vi "FOCUS_V42_H37.vi"(9 "X-pixels":sgl=256.0, 11 "Run":bool) -> (0 "Retrace pixels":sgl, 10 "Pixel Clock (Hz)":sgl)   [LabVIEW 2010] (continued)
                n477 = Add(x=w2194, y="x jog") -> (x+y=w2189:dbl[])
                n478 = And(x=w2108, y=TRUE ("XScale")) -> (x .and. y?=w2107:bool)
                n479 = Delete From Array(array=w2145, length=w2140, index=0) -> (deleted portion=w2143:dbl[], array with subset deleted=w2142:dbl[])
                n480 = Build Array (concatenate)(w2142, w2143) -> (w2112:dbl[])
                n481 = case shown="False" w2110 {
                  tunnel: w2189 -> [w2216 w2220]
                  tunnel: w2185 -> [w2215 w2219]
                  tunnel: [w2214 w2217] -> w2175
                  tunnel: w2112 -> [w2208 w2218]
                  frame False {
                    n482 = local read "Position piezo [µm]"() -> (w2212:sgl)
                    n483 = Multiply(x=sgl 40.0 ("y"), y=w2208) -> (x*y=w2209:dbl[])
                    n484 = Subtract(x=w2209, y=w2212) -> (x-y=w2207:dbl[])
                    n485 = local read "scattering length [µm]"() -> (w2210:sgl)
                    n486 = Divide(x=w2207, y=w2210) -> (x/y=w2206:dbl[])
                    n487 = local read "Intensity"() -> (w2213:sgl)
                    n488 = Exponential(1:w2206) -> (0:w2205:dbl[])
                    n489 = Multiply(x=w2205, y=w2213) -> (x*y=w2204:dbl[])
                    n490 = Build Array(w2216, w2215, w2208, w2204) -> (w2214:dbl[][])
                  }
                  frame True {
                    n491 = Build Array(w2220, w2219, w2218) -> (w2217:dbl[][])
                  }
                }
                n492 = case shown="True" w2110 {
                  tunnel: w2190 -> [_ w2263]
                  tunnel: [w2254 w2256] -> w2188
                  tunnel: [w2255 w2257] -> w2187
                  tunnel: w2175 -> [w2255 w2258]
                  frame False {
                    n493 = local read "total pixels in frame"() -> (w2254:sgl)
                  }
                  frame True {
                    n494 = local read "Scan Block Length"() -> (w2262:sgl)
                    n495 = Multiply(x=w2262, y=w2263) -> (x*y=w2261:sgl)
                    n496 = Multiply(x=w2261, y=1.0) -> (x*y=w2256:dbl)
                    n497 = Initialize Array(0.0 ("element"), 2 ("dimension size"), w2256) -> ()  [unwired: 1 out]
                    n498 = Array Subset(array=w2258, length (col)=w2256) -> (w2257:dbl[][])  [unwired: 3 in]
                  }
                }
                "y scan signals" <- w2169
                "x scan signals" <- w2170
              }
              frame 1 {
                n499 = local read "[µm] per pixel at zoom 1"() -> (w2305:sgl)
                n500 = local read "Y-lines"() -> (w2304:sgl)
                n501 = local read "Rotation z"() -> (w2280:sgl)
                n502 = local read "On?"() -> (w2281:bool)
                n503 = local read "Scanner dead time"() -> (w2297:sgl)
                n504 = case shown="False" w2281 {
                  tunnel: w2280 -> [_ w2420]
                  tunnel: [sgl 0.0 ("Rotation z") w2420] -> w2279
                  frame False {
                  }
                  frame True {
                  }
                }
                n505 = Divide(x=w2279, y=360.0) -> (x/y=w2351:dbl)
                n506 = Multiply(x=w2351, y=6.283185307179586) -> (x*y=w2349:dbl)
                n507 = Build Array(w2355, w2354, w2353) -> (w2335:dbl[][])
                n508 = Divide(x=w2297, y=w2292) -> (x/y=w2299:sgl)
                n509 = Sine(x=w2349) -> (sin(x)=w2308:dbl)
                n510 = Cosine(x=w2349) -> (cos(x)=w2348:dbl)
                n511 = Multiply(x=w2305, y=w2304) -> (x*y=w2302:sgl)
                n512 = Add(x=sgl 2.0, y=w2299) -> (x+y=w2298:sgl)
                n513 = Negate(x=w2308) -> (-x=w2347:dbl)
                n514 = Array Subset(array=w2335, length (row)=1 ("length")) -> (w2338:dbl[][])  [unwired: 3 in]
                n515 = Array Subset(array=w2335, index (row)=1 ("index")) -> (w2342:dbl[][])  [unwired: 3 in]
                n516 = local read "Zoom"() -> (w2309:sgl)
                n517 = Build Array(w2308, w2348) -> (w2344:dbl[])
                n518 = Build Array(w2348, w2347) -> (w2345:dbl[])
                n519 = local read "total y pixels"() -> (w2294:sgl)
                n520 = Round To Nearest(number=w2298) -> (nearest integer value=w2296:sgl)
                n521 = Build Array(w2345, w2344) -> (w2343:dbl[][])
                n522 = local read "Rotation"() -> (w2359:sgl)
                n523 = call-poly <vilib>:"A x B.vi"("B"=w2342, "A"=w2343) -> ("A x B"=w2336:T15)  [unwired: 1 out]
                n524 = local read "Position piezo [µm]"() -> (w2307:sgl)
                n525 = Divide(x=w2302, y=w2309) -> (x/y=w2313:sgl)
                n526 = local read "x-step (um)"() -> (w2286:sgl)
                n527 = local read "y-step (um)"() -> (w2287:sgl)
                n528 = local read "z-step (um)"() -> (w2301:sgl)
                n529 = local read "total x pixels"() -> (w2295:sgl)
                n530 = Divide(x=w2313, y=sgl 40.0) -> (x/y=w2319:sgl)
                n531 = Multiply(x=w2359, y=-1.0) -> (x*y=w2362:dbl)
                n532 = Index Array(array=w2336, index (row)=0 ("disabled index (col)")) -> (element=w2337:dbl[])  [unwired: 1 in]
                n533 = Index Array(array=w2336, index (row)=1 ("disabled index (col)")) -> (element=w2310:dbl[])  [unwired: 1 in]
                n534 = Array Max & Min(array=w2310) -> (max value=w2311:dbl, min value=w2316:dbl)  [unwired: 2 out]
                n535 = Subtract(x=w2311, y=w2316) -> (x-y=w2318:dbl)
                n536 = local read "Mode selector"() -> (w2273:u16)
                n537 = Equal To 0?(x=w2318) -> (x = 0?=w2321:bool)
                n538 = Subtract(x=w2310, y=w2316) -> (x-y=w2322:dbl[])
                n539 = Subtract(x=w2362, y=360.0) -> (x-y=w2360:dbl)
                n540 = Multiply(x=w2319, y=w2308) -> (x*y=w2320:dbl)
                n541 = Divide(x=w2360, y=360.0) -> (x/y=w2368:dbl)
                n542 = Build Array (concatenate)(w2338, w2337) -> (w2334:dbl[][])
                n543 = Equal To 0?(x=w2286) -> (x = 0?=w2285:bool)
                n544 = Equal To 0?(x=w2287) -> (x = 0?=w2284:bool)
                n545 = Equal To 0?(x=w2301) -> (x = 0?=w2283:bool)
                n546 = Divide(x=w2307, y=sgl 40.0) -> (x/y=w2303:sgl)
                n547 = case shown="False" w2321 {
                  tunnel: [w2448 w2449] -> w2317
                  tunnel: w2318 -> [w2447 _]
                  tunnel: w2320 -> [w2445 _]
                  tunnel: w2303 -> [w2443 w2451]
                  tunnel: w2322 -> [w2437 w2450]
                  frame False {
                    n548 = Divide(x=w2437, y=w2447) -> (x/y=w2446:dbl[])
                    n549 = Multiply(x=w2446, y=w2445) -> (x*y=w2444:dbl[])
                    n550 = Add(x=w2444, y=w2443) -> (x+y=w2436:dbl[])
                    n551 = Array Max & Min(array=w2436) -> (max value=w2442:dbl, min value=w2439:dbl)  [unwired: 2 out]
                    n552 = Subtract(x=w2442, y=w2439) -> (x-y=w2441:dbl)
                    n553 = Divide(x=w2441, y=2.0) -> (x/y=w2438:dbl)
                    n554 = Subtract(x=w2436, y=w2438) -> (x-y=w2448:dbl[])
                  }
                  frame True {
                    n555 = Add(x=w2450, y=w2451) -> (x+y=w2449:dbl[])
                  }
                }
                n556 = Multiply(x=w2368, y=6.283185307179586) -> (x*y=w2370:dbl)
                n557 = Compound Arithmetic op=AND(w2285, w2284, w2283) -> (w2282:bool)
                n558 = Equal?(x=w2273, y=u16 4) -> (x = y?=w2266:bool)
                n559 = Sine(x=w2370) -> (sin(x)=w2374:dbl)
                n560 = Cosine(x=w2370) -> (cos(x)=w2375:dbl)
                n561 = case shown="False" w2282 {
                  tunnel: [w2428 w2435] -> w2293
                  tunnel: w2296 -> [w2423 w2431]
                  frame True {
                    w2427 = 10178 items=["Finite Samples"=10178, "Continuous Samples"=10123, "Hardware Timed Single Point"=12522] ("sample mode")
                    n562 = local read "total pixels in frame"() -> (w2425:sgl)
                    n563 = local read "Number of frames"() -> (w2424:sgl)
                    n564 = local read "Averaging"() -> (w2426:u16)
                    n565 = Compound Arithmetic op=MULTIPLY(w2426, w2424, w2425) -> (w2422:sgl)
                    n566 = Add(x=w2422, y=w2423) -> (x+y=w2421:sgl)
                    n567 = Bundle(w2421, "sample mode"=w2427) -> (w2428:cluster{sgl, "sample mode":i32})  [unwired: 1 in]
                  }
                  frame False {
                    w2434 = 10178 items=["Finite Samples"=10178, "Continuous Samples"=10123, "Hardware Timed Single Point"=12522] ("sample mode")
                    n568 = local read "total pixels in frame"() -> (w2432:sgl)
                    n569 = local read "Averaging"() -> (w2433:u16)
                    n570 = Compound Arithmetic op=MULTIPLY(w2433, w2432) -> (w2430:sgl)
                    n571 = Add(x=w2430, y=w2431) -> (x+y=w2429:sgl)
                    n572 = Bundle(w2429, "sample mode"=w2434) -> (w2435:cluster{sgl, "sample mode":i32})  [unwired: 1 in]
                  }
                }
                n573 = Negate(x=w2374) -> (-x=w2371:dbl)
                n574 = local read "FocusModeSelector"() -> (w2277:bool)
                n575 = Build Array(w2375, w2371) -> (w2372:dbl[])
                n576 = Build Array(w2374, w2375) -> (w2373:dbl[])
                n577 = Build Array(w2372, w2373) -> (w2358:dbl[][])
                n578 = call-poly <vilib>:"A x B.vi"("B"=w2334, "A"=w2358) -> ("A x B"=w2333:T15)  [unwired: 1 out]
                n579 = In Range and Coerce(upper limit=0.0 ("element"), x=w2317, lower limit=10.0 ("element")) -> (coerced(x)=w2330:dbl[])  [unwired: 1 out]
                n580 = Divide(x=w2333, y=w2309) -> (x/y=w2332:T15)
                n581 = Array Size(array=w2330) -> (size(s)=w2329:i32)
                n582 = local read "x jog"() -> (w2290:sgl)
                n583 = local read "y jog"() -> (w2289:sgl)
                n584 = case shown="True" w2277 {
                  tunnel: w2268 -> [w2410 w2418]
                  tunnel: [w2409 w2417] -> w2267
                  tunnel: w2269 -> [w2408 w2416]
                  frame True {
                    n585 = Concatenate Strings(w2408, tag "/ao0," ("physical channels"), w2408, tag "/ao1," ("physical channels"), w2408, tag "/ao2" ("physical channels")) -> (w2405:string)
                    n586 = Type Cast(type=w2410, x=w2405) -> (*(type *) &x=w2409:tag)
                  }
                  frame False {
                    n587 = Concatenate Strings(w2416, tag "/ao0," ("physical channels"), w2416, tag "/ao1," ("physical channels"), w2416, tag "/ao2," ("physical channels"), w2416, tag "/ao3" ("physical channels")) -> (w2413:string)
                    n588 = Type Cast(type=w2418, x=w2413) -> (*(type *) &x=w2417:tag)
                  }
                }
                n589 = case shown="True" w2266 {
                  tunnel: w2268 -> [w2381 _]
                  tunnel: [w2380 w2382] -> w2265
                  tunnel: w2269 -> [w2379 _]
                  tunnel: w2267 -> [_ w2382]
                  frame True {
                    n590 = Concatenate Strings(w2379, tag "/ao0," ("physical channels"), w2379, tag "/ao1" ("physical channels")) -> (w2376:string)
                    n591 = Type Cast(type=w2381, x=w2376) -> (*(type *) &x=w2380:tag)
                  }
                  frame False {
                  }
                }
                n592 = Index Array(array=w2332, index (row)=0 ("disabled index (col)")) -> (element=w2366:dbl[])  [unwired: 1 in]
                n593 = Index Array(array=w2332, index (row)=1 ("disabled index (col)")) -> (element=w2365:dbl[])  [unwired: 1 in]
                n594 = Multiply(x=w2329, y=15) -> (x*y=w2324:i32)
                n595 = local read "total pixels in frame"() -> (w2291:sgl)
                n596 = Divide(x=w2324, y=360.0) -> (x/y=w2325:dbl)
                n597 = Add(x=w2365, y=w2289) -> (x+y=w2274:dbl[])
                n598 = Add(x=w2366, y=w2290) -> (x+y=w2275:dbl[])
                n599 = Not(x=w2277) -> (.not. x?=w2276:bool)
                n600 = Delete From Array(array=w2330, length=w2325, index=0) -> (deleted portion=w2328:dbl[], array with subset deleted=w2327:dbl[])
                n601 = Build Array (concatenate)(w2327, w2328) -> (w2278:dbl[])
                n602 = case shown="False" w2277 {
                  tunnel: w2275 -> [w2399 w2403]
                  tunnel: w2274 -> [w2398 w2402]
                  tunnel: [w2397 w2400] -> w2271
                  tunnel: w2278 -> [w2394 w2401]
                  frame False {
                    n603 = local read "Position piezo [µm]"() -> (w2389:sgl)
                    n604 = Multiply(x=sgl 40.0 ("y"), y=w2394) -> (x*y=w2395:dbl[])
                    n605 = Subtract(x=w2395, y=w2389) -> (x-y=w2393:dbl[])
                    n606 = local read "scattering length [µm]"() -> (w2388:sgl)
                    n607 = Divide(x=w2393, y=w2388) -> (x/y=w2392:dbl[])
                    n608 = Exponential(1:w2392) -> (0:w2391:dbl[])
                    n609 = local read "Intensity"() -> (w2387:sgl)
                    n610 = Multiply(x=w2391, y=w2387) -> (x*y=w2390:dbl[])
                    n611 = Build Array(w2399, w2398, w2394, w2390) -> (w2397:dbl[][])
                  }
                  frame True {
                    n612 = Build Array(w2403, w2402, w2401) -> (w2400:dbl[][])
                  }
                }
                n613 = case shown="False" w2266 {
                  tunnel: w2275 -> [_ w2386]
                  tunnel: w2274 -> [_ w2385]
                  tunnel: w2271 -> [w2383 _]
                  tunnel: [w2383 w2384] -> w2270
                  frame False {
                  }
                  frame True {
                    n614 = Build Array(w2386, w2385) -> (w2384:dbl[][])
                  }
                }
              }
              frame 2 {
                w2466 = 10123 items=["Finite Samples"=10178, "Continuous Samples"=10123, "Hardware Timed Single Point"=12522] ("sample mode")
                n615 = local read "[µm] per pixel at zoom 1"() -> (w2473:sgl)
                n616 = local read "Y-lines"() -> (w2472:sgl)
                n617 = local read "Rotation z"() -> (w2453:sgl)
                n618 = local read "On?"() -> (w2454:bool)
                n619 = case shown="False" w2454 {
                  tunnel: w2453 -> [_ w2553]
                  tunnel: [sgl 0.0 ("Rotation z") w2553] -> w2452
                  frame False {
                  }
                  frame True {
                  }
                }
                n620 = Divide(x=w2452, y=360.0) -> (x/y=w2520:dbl)
                n621 = case shown="False" "Linescan mode" {
                  tunnel: w2459 -> [w2555 _]
                  tunnel: [w2555 w2558] -> w2458
                  tunnel: [w2554 w2559] -> w2457
                  tunnel: w2456 -> [_ w2559]
                  frame False {
                    n622 = Array Size(array=w2555) -> (size(s)=w2556:i32)
                    n623 = Initialize Array(0.0 ("element"), w2556) -> (w2554:dbl[])
                  }
                  frame True {
                    n624 = Array Size(array=w2559) -> (size(s)=w2560:i32)
                    n625 = Initialize Array(0.0 ("element"), w2560) -> (w2558:dbl[])
                  }
                }
                n626 = Multiply(x=w2520, y=6.283185307179586) -> (x*y=w2518:dbl)
                n627 = Build Array(w2458, w2457, w2522) -> (w2504:dbl[][])
                n628 = Sine(x=w2518) -> (sin(x)=w2476:dbl)
                n629 = Cosine(x=w2518) -> (cos(x)=w2517:dbl)
                n630 = Multiply(x=w2473, y=w2472) -> (x*y=w2470:sgl)
                n631 = Negate(x=w2476) -> (-x=w2516:dbl)
                n632 = Array Subset(array=w2504, length (row)=1 ("length")) -> (w2507:dbl[][])  [unwired: 3 in]
                n633 = Array Subset(array=w2504, index (row)=1 ("index")) -> (w2511:dbl[][])  [unwired: 3 in]
                n634 = local read "Zoom"() -> (w2478:sgl)
                n635 = Build Array(w2476, w2517) -> (w2513:dbl[])
                n636 = Build Array(w2517, w2516) -> (w2514:dbl[])
                n637 = local read "total y pixels"() -> (w2464:sgl)
                n638 = Build Array(w2514, w2513) -> (w2512:dbl[][])
                n639 = local read "Rotation"() -> (w2533:sgl)
                n640 = local read "total x pixels"() -> (w2463:sgl)
                n641 = call-poly <vilib>:"A x B.vi"("B"=w2511, "A"=w2512) -> ("A x B"=w2505:T15)  [unwired: 1 out]
                n642 = local read "Position piezo [µm]"() -> (w2475:sgl)
                n643 = Divide(x=w2470, y=w2478) -> (x/y=w2482:sgl)
                n644 = Divide(x=w2482, y=sgl 40.0) -> (x/y=w2488:sgl)
                n645 = Multiply(x=w2533, y=-1.0) -> (x*y=w2536:dbl)
                n646 = Index Array(array=w2505, index (row)=0 ("disabled index (col)")) -> (element=w2506:dbl[])  [unwired: 1 in]
                n647 = Index Array(array=w2505, index (row)=1 ("disabled index (col)")) -> (element=w2479:dbl[])  [unwired: 1 in]
                n648 = Array Max & Min(array=w2479) -> (max value=w2480:dbl, min value=w2485:dbl)  [unwired: 2 out]
                n649 = Subtract(x=w2480, y=w2485) -> (x-y=w2487:dbl)
                n650 = Equal To 0?(x=w2487) -> (x = 0?=w2490:bool)
                n651 = Subtract(x=w2479, y=w2485) -> (x-y=w2491:dbl[])
                n652 = Subtract(x=w2536, y=360.0) -> (x-y=w2534:dbl)
                n653 = Multiply(x=w2488, y=w2476) -> (x*y=w2489:dbl)
                n654 = Divide(x=w2534, y=360.0) -> (x/y=w2544:dbl)
                n655 = Build Array (concatenate)(w2507, w2506) -> (w2503:dbl[][])
                n656 = Divide(x=w2475, y=sgl 40.0) -> (x/y=w2471:sgl)
                n657 = case shown="False" w2490 {
                  tunnel: [w2574 w2575] -> w2486
                  tunnel: w2487 -> [w2573 _]
                  tunnel: w2489 -> [w2571 _]
                  tunnel: w2471 -> [w2569 w2577]
                  tunnel: w2491 -> [w2563 w2576]
                  frame False {
                    n658 = Divide(x=w2563, y=w2573) -> (x/y=w2572:dbl[])
                    n659 = Multiply(x=w2572, y=w2571) -> (x*y=w2570:dbl[])
                    n660 = Add(x=w2570, y=w2569) -> (x+y=w2562:dbl[])
                    n661 = Array Max & Min(array=w2562) -> (max value=w2568:dbl, min value=w2565:dbl)  [unwired: 2 out]
                    n662 = Subtract(x=w2568, y=w2565) -> (x-y=w2567:dbl)
                    n663 = Divide(x=w2567, y=2.0) -> (x/y=w2564:dbl)
                    n664 = Subtract(x=w2562, y=w2564) -> (x-y=w2574:dbl[])
                  }
                  frame True {
                    n665 = Add(x=w2576, y=w2577) -> (x+y=w2575:dbl[])
                  }
                }
                n666 = Multiply(x=w2544, y=6.283185307179586) -> (x*y=w2546:dbl)
                n667 = Sine(x=w2546) -> (sin(x)=w2550:dbl)
                n668 = Cosine(x=w2546) -> (cos(x)=w2551:dbl)
                n669 = Negate(x=w2550) -> (-x=w2547:dbl)
                n670 = Build Array(w2551, w2547) -> (w2548:dbl[])
                n671 = Build Array(w2550, w2551) -> (w2549:dbl[])
                n672 = Bundle("sample mode"=w2466, "sample mode"=w2466) -> (w2462:cluster{"sample mode":i32, "sample mode":i32})  [unwired: 1 in]
                n673 = Build Array(w2548, w2549) -> (w2532:dbl[][])
                n674 = call-poly <vilib>:"A x B.vi"("B"=w2503, "A"=w2532) -> ("A x B"=w2502:T15)  [unwired: 1 out]
                n675 = In Range and Coerce(upper limit=0.0 ("element"), x=w2486, lower limit=10.0 ("element")) -> (coerced(x)=w2499:dbl[])  [unwired: 1 out]
                n676 = Divide(x=w2502, y=w2478) -> (x/y=w2501:T15)
                n677 = Array Size(array=w2499) -> (size(s)=w2498:i32)
                n678 = local read "x jog"() -> (w2468:sgl)
                n679 = local read "y jog"() -> (w2467:sgl)
                n680 = Index Array(array=w2501, index (row)=0 ("disabled index (col)")) -> (element=w2542:dbl[])  [unwired: 1 in]
                n681 = Index Array(array=w2501, index (row)=1 ("disabled index (col)")) -> (element=w2541:dbl[])  [unwired: 1 in]
                n682 = Multiply(x=w2498, y=15) -> (x*y=w2493:i32)
                n683 = Divide(x=w2493, y=360.0) -> (x/y=w2494:dbl)
                n684 = Add(x=w2541, y=w2467) -> (x+y=w2538:dbl[])
                n685 = Multiply(x=w2463, y=sgl 1.0) -> (x*y=w2461:sgl)
                n686 = Add(x=w2542, y=w2468) -> (x+y=w2540:dbl[])
                n687 = Delete From Array(array=w2499, length=w2494, index=0) -> (deleted portion=w2497:dbl[], array with subset deleted=w2496:dbl[])
                n688 = Concatenate Strings(w2528, tag "/ao0," ("physical channels"), w2528, tag "/ao1," ("physical channels"), w2528, tag "/ao2" ("physical channels")) -> (w2524:string)
                n689 = Build Array (concatenate)(w2496, w2497) -> (w2477:dbl[])
                n690 = Build Array(w2540, w2538, w2477) -> (w2469:dbl[][])
                n691 = Type Cast(type=w2529, x=w2524) -> (*(type *) &x=w2527:tag)
              }
              frame 3 {
                w2582 = 10123 items=["Finite Samples"=10178, "Continuous Samples"=10123, "Hardware Timed Single Point"=12522] ("sample mode")
                n692 = case shown="True" w2592 {
                  tunnel: w2596 -> [_ _]
                  tunnel: [w2600 w2619] -> w2591
                  tunnel: [w2602 w2637] -> w2595
                  tunnel: [w2601 w2614] -> w2594
                  tunnel: [w2601 w2614] -> w2593
                  tunnel: w2580 -> [_ w2611]
                  tunnel: w2579 -> [_ w2607]
                  frame False {
                    n693 = local read "Y-lines FreeLine"() -> (w2602:sgl)
                    n694 = local read "X-pixels FreeLine"() -> (w2601:sgl)
                    n695 = local read "y scan signals"() -> (w2597:dbl[])
                    n696 = Array Max & Min(array=w2597) -> (max value=w2599:dbl, min value=w2598:dbl)  [unwired: 2 out]
                    n697 = property on="XY Graph 1" class="XYGraph (strict)"("X Scale.Range:Maximum"=w2599, "X Scale.Range:Minimum"=w2598, "Y Scale.Range:Maximum"=w2599, "Y Scale.Range:Minimum"=w2598) -> ()  [unwired: 2 in, 2 out]
                    n698 = property on="XY Graph 2" class="XYGraph (strict)"("X Scale.Range:Maximum"=w2599, "X Scale.Range:Minimum"=w2598, "Y Scale.Range:Maximum"=w2599, "Y Scale.Range:Minimum"=w2598) -> ()  [unwired: 2 in, 2 out]
                    n699 = local read "ScanLineFreeLine"() -> (w2600:sgl[][])
                  }
                  frame True {
                    w2655 = 1 ("length")
                    # "Rotation"
                    n700 = local read "Scan Cut-Off (either end)"() -> (w2604:sgl)
                    n701 = Index Array(array=w2607, index=w2604) -> (element=w2610:dbl)
                    n702 = local read "X-pixels"() -> (w2606:sgl)
                    n703 = local read "Y-lines"() -> (w2605:sgl)
                    n704 = property on="XY Graph 2" class="XYGraph (strict)"("Visible"=TRUE) -> ()  [unwired: 2 in, 2 out]
                    n705 = property on="XY Graph 1" class="XYGraph (strict)"("Visible"=TRUE) -> ()  [unwired: 2 in, 2 out]
                    n706 = Divide(x=w2606, y=w2605) -> (x/y=w2609:sgl)
                    n707 = property on="Image 2" class="IntGraph (strict)"() -> ("Color Table"=w2645:u32[])  [unwired: 2 in, 2 out]
                    n708 = Divide(x=w2610, y=w2609) -> (x/y=w2608:dbl)
                    n709 = Absolute Value(x=w2608) -> (abs(x)=w2603:dbl)
                    n710 = local read "Image 2"() -> (w2670:u8[][])
                    n711 = local read "Image 1"() -> (w2669:u8[][])
                    n712 = local read "X-pixels"() -> (w2634:sgl)
                    n713 = local read "Y-lines"() -> (w2633:sgl)
                    n714 = call "FreeLine2D.vi"("Color Table"=w2645, "data channel 2"=w2670, "X-pixels"=w2634, "Y-lines"=w2633, "data channel"=w2669) -> ("user defined lines"=w2637:i16, "PointsCoordinates"=w2639:i32[][], "pixel x"=w2636:dbl[], "pixel y"=w2635:dbl[], "number of pixels"=w2614:dbl, "Pixel Clock (Hz)"=w2613:dbl)
                    "X-pixels FreeLine" <- w2614
                    "Pixel Clock (Hz) FreeLine" <- w2613
                    n715 = local write "Y-lines FreeLine"(w2637) -> ()
                    n716 = Array Max & Min(array=w2611) -> (max value=w2618:dbl, min value=w2617:dbl)  [unwired: 2 out]
                    n717 = call "CalcxyscansignalsudlFOCUS.vi"("Y-Lines"=w2633, "X Pixels"=w2634, "MaxValuey"=w2603, "MaxValuex"=w2603, "pixel y"=w2635, "pixel x"=w2636) -> ("Signal y"=w2631:dbl[], "Signal x"=w2632:dbl[])
                    n718 = Index Array(array=w2639, index (col)=0 ("disabled index (col)")) -> (element=w2643:i32[])  [unwired: 1 in]
                    n719 = Index Array(array=w2639, index (col)=1 ("disabled index (col)")) -> (element=w2642:i32[])  [unwired: 1 in]
                    n720 = local write "new FreeLine?"(FALSE ("new udl?")) -> ()
                    n721 = Bundle("PointsCoordinates"=w2643, "PointsCoordinates"=w2642) -> (w2638:T16)  [unwired: 1 in]
                    n722 = local read "Rotation"() -> (w2627:sgl)
                    n723 = property on="XY Graph 1" class="XYGraph (strict)"("X Scale.Range:Maximum"=w2618, "X Scale.Range:Minimum"=w2617, "Y Scale.Range:Maximum"=w2618, "Y Scale.Range:Minimum"=w2617) -> ()  [unwired: 2 in, 2 out]
                    n724 = Build Array(w2632, w2631) -> (w2624:dbl[][])
                    n725 = Multiply(x=w2627, y=-1.0) -> (x*y=w2629:dbl)
                    n726 = local write "Histogram1"(w2638) -> ()
                    n727 = local write "Histogram2"(w2638) -> ()
                    n728 = Subtract(x=w2629, y=360.0) -> (x-y=w2626:dbl)
                    n729 = local read "Zoom"() -> (w2652:sgl)
                    n730 = Divide(x=w2626, y=360.0) -> (x/y=w2678:dbl)
                    n731 = property on="XY Graph 2" class="XYGraph (strict)"("X Scale.Range:Maximum"=w2618, "X Scale.Range:Minimum"=w2617, "Y Scale.Range:Maximum"=w2618, "Y Scale.Range:Minimum"=w2617) -> ()  [unwired: 2 in, 2 out]
                    n732 = Multiply(x=w2678, y=6.283185307179586) -> (x*y=w2676:dbl)
                    n733 = Divide(x=w2624, y=w2652) -> (x/y=w2623:dbl[][])
                    n734 = Reciprocal(x=w2613) -> (1/x=w2616:dbl)
                    n735 = property on="XY Graph 3" class="XYGraph (strict)"("X Scale.Range:Maximum"=w2618, "X Scale.Range:Minimum"=w2617, "Y Scale.Range:Maximum"=w2618, "Y Scale.Range:Minimum"=w2617) -> ()  [unwired: 2 in, 2 out]
                    n736 = Sine(x=w2676) -> (sin(x)=w2672:dbl)
                    n737 = Cosine(x=w2676) -> (cos(x)=w2671:dbl)
                    n738 = Negate(x=w2672) -> (-x=w2675:dbl)
                    n739 = Multiply(x=w2616, y=sgl 1000000.0) -> (x*y=w2612:dbl)
                    n740 = Array Subset(array=w2632, index=0, length=1) -> (w2662:dbl[])
                    n741 = Array Subset(array=w2631, index=0, length=1) -> (w2661:dbl[])
                    n742 = local write "pixel dwell time [us] FreeLine"(w2612) -> ()
                    n743 = Build Array(w2671, w2675) -> (w2674:dbl[])
                    n744 = Build Array(w2672, w2671) -> (w2673:dbl[])
                    n745 = property on="XY Graph 4" class="XYGraph (strict)"("X Scale.Range:Maximum"=w2618, "X Scale.Range:Minimum"=w2617, "Y Scale.Range:Maximum"=w2618, "Y Scale.Range:Minimum"=w2617) -> ()  [unwired: 2 in, 2 out]
                    n746 = Bundle("Signal x"=w2632, "Signal y"=w2631) -> (w2660:cluster{"Signal x":dbl[], "Signal y":dbl[]})  [unwired: 1 in]
                    n747 = Bundle(w2662, w2661) -> (w2659:cluster{dbl[], dbl[]})  [unwired: 1 in]
                    n748 = Build Array(w2674, w2673) -> (w2625:dbl[][])
                    n749 = Decrement(x=w2614) -> (x-1=w2654:dbl)
                    n750 = Array Subset(array=w2632, index=w2654, length=w2655) -> (w2656:dbl[])
                    n751 = Array Subset(array=w2631, index=w2654, length=w2655) -> (w2657:dbl[])
                    n752 = call-poly <vilib>:"A x B.vi"("B"=w2623, "A"=w2625) -> ("A x B"=w2622:T15)  [unwired: 1 out]
                    n753 = Bundle(w2656, w2657) -> (w2653:cluster{dbl[], dbl[]})  [unwired: 1 in]
                    n754 = local read "x jog"() -> (w2646:sgl)
                    n755 = Index Array(array=w2622, index (row)=0 ("disabled index (col)")) -> (element=w2651:dbl[])  [unwired: 1 in]
                    n756 = Index Array(array=w2622, index (row)=1 ("disabled index (col)")) -> (element=w2650:dbl[])  [unwired: 1 in]
                    n757 = Build Array(w2660, w2659, w2653) -> (→"XY Graph 1" →"XY Graph 2":cluster{"Signal x":dbl[], "Signal y":dbl[]}[])
                    n758 = local read "y jog"() -> (w2647:sgl)
                    n759 = Add(x=w2650, y=w2647) -> (x+y=w2648:dbl[])
                    n760 = Add(x=w2651, y=w2646) -> (x+y=w2649:dbl[])
                    n761 = Build Array(w2649, w2648) -> (w2619:dbl[][])
                    "ScanLineFreeLine" <- w2619
                  }
                }
                n762 = Bundle("sample mode"=w2582, "sample mode"=w2582) -> (w2581:cluster{"sample mode":i32, "sample mode":i32})  [unwired: 1 in]
                n763 = local write "XScale"(TRUE ("XScale")) -> ()
                n764 = Concatenate Strings(w2586, tag "/ao0," ("physical channels"), w2586, tag "/ao1" ("physical channels")) -> (w2588:string)
                n765 = Type Cast(type=w2585, x=w2588) -> (*(type *) &x=w2584:tag)
              }
              frame 4 {
                w2686 = 10123 items=["Finite Samples"=10178, "Continuous Samples"=10123, "Hardware Timed Single Point"=12522] ("sample mode")
                n766 = case shown="True" w2695 {
                  tunnel: [w2731 w2783] -> w2701
                  tunnel: [w2730 w2746] -> w2697
                  tunnel: w2700 -> [_ _]
                  tunnel: [w2706 w2755] -> w2699
                  tunnel: [w2730 w2746] -> w2698
                  tunnel: w2684 -> [_ w2749]
                  tunnel: w2683 -> [_ w2748]
                  tunnel: w2682 -> [_ w2739]
                  tunnel: w2681 -> [_ w2738]
                  frame False {
                    n767 = local read "Zsin3D"() -> (w2714:sgl[])
                    n768 = local read "Amplitude Factor"() -> (w2712:sgl)
                    n769 = local read "y scan signals"() -> (w2720:dbl[])
                    n770 = Array Size(array=w2714) -> (size(s)=w2719:i32)
                    n771 = Add Array Elements(numeric array=w2714) -> (sum=w2718:sgl)
                    n772 = Divide(x=w2718, y=w2719) -> (x/y=w2715:sgl)
                    n773 = Subtract(x=w2714, y=w2715) -> (x-y=w2717:sgl[])
                    n774 = Multiply(x=w2717, y=w2712) -> (x*y=w2716:sgl[])
                    n775 = local read "phase shift [°]"() -> (w2723:sgl)
                    n776 = Array Max & Min(array=w2720) -> (max value=w2722:dbl, min value=w2721:dbl)  [unwired: 2 out]
                    n777 = Add(x=w2716, y=w2715) -> (x+y=w2713:sgl[])
                    n778 = local read "Y-lines FreeLine"() -> (w2731:sgl)
                    n779 = local read "X-pixels FreeLine"() -> (w2730:sgl)
                    n780 = property on="XY Graph 1" class="XYGraph (strict)"("X Scale.Range:Maximum"=w2722, "X Scale.Range:Minimum"=w2721, "Y Scale.Range:Maximum"=w2722, "Y Scale.Range:Minimum"=w2721) -> ()  [unwired: 2 in, 2 out]
                    n781 = Array Size(array=w2713) -> (size(s)=w2707:i32)
                    n782 = Multiply(x=w2707, y=w2723) -> (x*y=w2728:sgl)
                    n783 = Divide(x=w2728, y=360.0) -> (x/y=w2727:dbl)
                    n784 = property on="XY Graph 2" class="XYGraph (strict)"("X Scale.Range:Maximum"=w2722, "X Scale.Range:Minimum"=w2721, "Y Scale.Range:Maximum"=w2722, "Y Scale.Range:Minimum"=w2721) -> ()  [unwired: 2 in, 2 out]
                    n785 = local read "Intensity"() -> (w2708:sgl)
                    n786 = local read "ZInt3D"() -> (w2709:sgl[])
                    n787 = Delete From Array(array=w2713, length=w2727, index=0) -> (deleted portion=w2724:sgl[], array with subset deleted=w2725:sgl[])
                    n788 = Build Array (concatenate)(w2725, w2724) -> (w2711:sgl[])
                    n789 = Multiply(x=w2709, y=w2708) -> (x*y=w2703:sgl[])
                    n790 = Initialize Array(w2708, w2707) -> ()  [unwired: 1 out]
                    n791 = property on="Histogram1" class="XYGraph (strict)"("Visible"=FALSE) -> ()  [unwired: 2 in, 2 out]
                    n792 = case shown="True" "Int Corr?" {
                      tunnel: w2703 -> [w2732 w2737]
                      tunnel: [w2732 w2736] -> w2702
                      frame False {
                      }
                      frame True {
                        n793 = local read "Image3Arrayd"() -> (w2733:u8[][])
                        n794 = call "NormalizeIntensityUDL3D.vi"("bigger"="Scale", "Image3Array"=w2733, "Pockel's cell original"=w2737, "File?"=FALSE) -> ("Pockel's cell corrected"=w2736:dbl[])
                      }
                    }
                    n795 = local read "ScanLineFreeLine"() -> (w2710:sgl[][])
                    n796 = Build Array (concatenate)(w2710, w2711, w2702) -> (w2706:dbl[][])
                  }
                  frame True {
                    w2821 = 1 ("length")
                    # "Rotation"
                    n797 = property on="Image 2" class="IntGraph (strict)"() -> ("Color Table"=w2792:u32[])  [unwired: 2 in, 2 out]
                    n798 = local read "Scan Cut-Off (either end)"() -> (w2801:sgl)
                    n799 = local write "new FreeLine?"(FALSE ("new 3D udl?")) -> ()
                    n800 = local read "pixelstoµm"() -> (w2813:sgl)
                    n801 = property on="XY Graph 2" class="XYGraph (strict)"("Visible"=TRUE) -> ()  [unwired: 2 in, 2 out]
                    n802 = property on="XY Graph 1" class="XYGraph (strict)"("Visible"=TRUE) -> ()  [unwired: 2 in, 2 out]
                    n803 = local read "Number of frames"() -> (w2817:sgl)
                    n804 = local read "X-pixels"() -> (w2803:sgl)
                    n805 = local read "Y-lines"() -> (w2802:sgl)
                    n806 = Index Array(array=w2739, index=w2801) -> (element=w2740:dbl)
                    n807 = Divide(x=w2803, y=w2802) -> (x/y=w2804:sgl)
                    n808 = local read "X-pixels"() -> (w2771:sgl)
                    n809 = local read "Y-lines"() -> (w2770:sgl)
                    n810 = Divide(x=w2740, y=w2804) -> (x/y=w2800:dbl)
                    n811 = local read "z-step (um)"() -> (w2818:sgl)
                    n812 = Absolute Value(x=w2800) -> (abs(x)=w2772:dbl)
                    n813 = local read "Zoom"() -> (w2814:sgl)
                    n814 = call "FreeLine3D.vi"("Data1"=w2749, "z step (µm)"=w2818, "Color Table"=w2792, "Y-lines"=w2770, "X-pixels"=w2771, "Data2"=w2748, "pixelstoµm"=w2813, "z planes"=w2817, "zoom"=w2814) -> ("user defined lines"=w2783:i16, "x-values [pixels]"=w2774:dbl[], "pockel's cell"=w2753:dbl[], "y-values [pixels]"=w2773:dbl[], "PointsCoordinates"=w2788:i32[][], "pixel clock [Hz]"=w2744:dbl, "z-values [µm]"=w2747:dbl[])
                    "Pixel Clock z (Hz) FreeLine" <- w2744
                    "PointsCoordinates" <- w2788
                    "ZInt3D" <- w2753
                    n815 = local write "Y-lines FreeLine"(w2783) -> ()
                    n816 = Divide(x=w2747, y=40.0) -> (x/y=w2779:dbl[])
                    "Zsin3D" <- w2779
                    n817 = Array Size(array=w2779) -> (size(s)=w2750:i32)
                    n818 = Add Array Elements(numeric array=w2779) -> (sum=w2782:dbl)
                    n819 = Divide(x=w2782, y=w2750) -> (x/y=w2777:dbl)
                    n820 = Subtract(x=w2779, y=w2777) -> (x-y=w2781:dbl[])
                    n821 = Multiply(x=w2781, y="Amplitude Factor") -> (x*y=w2778:dbl[])
                    n822 = Add(x=w2778, y=w2777) -> (x+y=w2776:dbl[])
                    n823 = Array Size(array=w2776) -> (size(s)=w2810:i32)
                    n824 = Array Size(array=w2747) -> (size(s)=w2746:i32)
                    n825 = Array Max & Min(array=w2738) -> (max value=w2791:dbl, min value=w2790:dbl)  [unwired: 2 out]
                    n826 = call "CalcxyscansignalsudlFOCUS.vi"("Y-Lines"=w2770, "X Pixels"=w2771, "MaxValuey"=w2772, "MaxValuex"=w2772, "pixel y"=w2773, "pixel x"=w2774) -> ("Signal y"=w2768:dbl[], "Signal x"=w2769:dbl[])
                    n827 = Multiply(x=w2810, y="phase shift [°]") -> (x*y=w2811:sgl)
                    n828 = Divide(x=w2811, y=360.0) -> (x/y=w2808:dbl)
                    n829 = local write "Pixel Clock (Hz) FreeLine"(w2744) -> ()
                    n830 = Delete From Array(array=w2776, length=w2808, index=0) -> (deleted portion=w2805:dbl[], array with subset deleted=w2806:dbl[])
                    n831 = Build Array(w2769, w2768) -> (w2761:dbl[][])
                    n832 = property on="XY Graph 1" class="XYGraph (strict)"("X Scale.Range:Maximum"=w2791, "X Scale.Range:Minimum"=w2790, "Y Scale.Range:Maximum"=w2791, "Y Scale.Range:Minimum"=w2790) -> ()  [unwired: 2 in, 2 out]
                    n833 = Build Array (concatenate)(w2806, w2805) -> (w2756:dbl[])
                    n834 = Index Array(array=w2788, index (col)=0 ("disabled index (col)")) -> (element=w2789:i32[])  [unwired: 1 in]
                    n835 = Index Array(array=w2788, index (col)=1 ("disabled index (col)")) -> (element=w2787:i32[])  [unwired: 1 in]
                    n836 = local read "Rotation"() -> (w2764:sgl)
                    n837 = local read "Intensity"() -> (w2752:sgl)
                    n838 = Multiply(x=w2764, y=-1.0) -> (x*y=w2766:dbl)
                    n839 = local read "Zoom"() -> (w2799:sgl)
                    n840 = property on="XY Graph 2" class="XYGraph (strict)"("X Scale.Range:Maximum"=w2791, "X Scale.Range:Minimum"=w2790, "Y Scale.Range:Maximum"=w2791, "Y Scale.Range:Minimum"=w2790) -> ()  [unwired: 2 in, 2 out]
                    n841 = Bundle("PointsCoordinates"=w2789, "PointsCoordinates"=w2787) -> (→"Histogram1" →"Histogram2":T16)  [unwired: 1 in]
                    n842 = Subtract(x=w2766, y=360.0) -> (x-y=w2763:dbl)
                    n843 = Divide(x=w2761, y=w2799) -> (x/y=w2760:dbl[][])
                    n844 = Reciprocal(x=w2744) -> (1/x=w2743:dbl)
                    n845 = Divide(x=w2763, y=360.0) -> (x/y=w2841:dbl)
                    n846 = Multiply(x=w2753, y=w2752) -> ()  [unwired: 1 out]
                    n847 = local write "X-pixels FreeLine"(w2746) -> ()
                    n848 = Multiply(x=w2841, y=6.283185307179586) -> (x*y=w2839:dbl)
                    n849 = Multiply(x=w2743, y=sgl 1000000.0) -> (x*y=→"pixel dwell time [us] FreeLine":dbl)
                    n850 = Sine(x=w2839) -> (sin(x)=w2835:dbl)
                    n851 = Cosine(x=w2839) -> (cos(x)=w2834:dbl)
                    n852 = local read "x jog"() -> (w2795:sgl)
                    n853 = Array Subset(array=w2769, index=0, length=1) -> (w2827:dbl[])
                    n854 = Array Subset(array=w2768, index=0, length=1) -> (w2826:dbl[])
                    n855 = Negate(x=w2835) -> (-x=w2838:dbl)
                    n856 = local read "y jog"() -> (w2794:sgl)
                    n857 = Bundle("Signal x"=w2769, "Signal y"=w2768) -> (w2825:cluster{"Signal x":dbl[], "Signal y":dbl[]})  [unwired: 1 in]
                    n858 = Bundle(w2827, w2826) -> (w2824:cluster{dbl[], dbl[]})  [unwired: 1 in]
                    n859 = Divide(x=w2744, y=w2746) -> (x/y=w2745:dbl)
                    n860 = Build Array(w2834, w2838) -> (w2837:dbl[])
                    n861 = Build Array(w2835, w2834) -> (w2836:dbl[])
                    n862 = Decrement(x=w2746) -> (x-1=w2820:i32)
                    n863 = local write "z frequency"(w2745) -> ()
                    n864 = Build Array(w2837, w2836) -> (w2762:dbl[][])
                    n865 = Initialize Array(w2752, w2750) -> (w2751:sgl[])
                    n866 = Array Subset(array=w2769, index=w2820, length=w2821) -> (w2822:dbl[])
                    n867 = Array Subset(array=w2768, index=w2820, length=w2821) -> (w2823:dbl[])
                    n868 = call-poly <vilib>:"A x B.vi"("B"=w2760, "A"=w2762) -> ("A x B"=w2759:T15)  [unwired: 1 out]
                    n869 = Index Array(array=w2759, index (row)=0 ("disabled index (col)")) -> (element=w2798:dbl[])  [unwired: 1 in]
                    n870 = Index Array(array=w2759, index (row)=1 ("disabled index (col)")) -> (element=w2797:dbl[])  [unwired: 1 in]
                    n871 = Add(x=w2797, y=w2794) -> (x+y=w2796:dbl[])
                    n872 = Add(x=w2798, y=w2795) -> (x+y=w2775:dbl[])
                    n873 = Build Array(w2775, w2796) -> (w2754:dbl[][])
                    n874 = local write "ScanLineFreeLine"(w2754) -> ()
                    n875 = Bundle(w2822, w2823) -> (w2819:cluster{dbl[], dbl[]})  [unwired: 1 in]
                    n876 = Build Array (concatenate)(w2754, w2756, w2751) -> (w2755:dbl[][])
                    n877 = Build Array(w2825, w2824, w2819) -> (w2815:cluster{"Signal x":dbl[], "Signal y":dbl[]}[])
                    n878 = local write "XY Graph 1"(w2815) -> ()
                    n879 = local write "XY Graph 2"(w2815) -> ()
                  }
                }
                n880 = Bundle("sample mode"=w2686, "sample mode"=w2686) -> (w2685:cluster{"sample mode":i32, "sample mode":i32})  [unwired: 1 in]
                n881 = Concatenate Strings(w2689, tag "/ao0," ("physical channels"), w2689, tag "/ao1," ("physical channels"), w2689, tag "/ao2," ("physical channels"), w2689, tag "/ao3" ("physical channels")) -> (w2691:string)
                n882 = Type Cast(type=w2688, x=w2691) -> (*(type *) &x=w2687:tag)
              }
            }
          }
          frame True {
            n883 = case shown="True" "NewScanpattern" {
              tunnel: [w2933 w2943] -> w2853
              tunnel: [w2925 w2934] -> w2851
              tunnel: [w2926 w2935] -> w2850
              tunnel: [w2931 w2940] -> w2849
              tunnel: [w2925 w2934] -> w2846
              frame False {
                n884 = local read "ParametersFScope"() -> (w2932:T7)
                n885 = local read "ScanLineFScope"() -> (w2933:sgl[][])
                n886 = Unbundle(w2932) -> ("X frequeny [Hz]"=w2927:i32, "Y frequency \n[Hz]"=w2931:i32, "frequeny Trim"=w2928:dbl, "Samples/s"=w2925:i32)  [unwired: 2 out]
                n887 = local write "Pixel Clock (Hz) FScope"(w2925) -> ()
                n888 = Divide(x=w2928, y=200.0) -> (x/y=w2929:dbl)
                n889 = Add(x=w2927, y=w2929) -> (x+y=w2926:dbl)
              }
              frame True {
                n890 = call "LissajousPatternFScope.vi"("f max Y [Hz]"="f max Y", "f min Y [Hz]"="f min Y", "f max X [Hz]"="f max X", "f min X [Hz]"="f min X") -> ("Parameters"=w2941:T7, "ScanData"=w2943:dbl[][])  [unwired: 1 out]
                "ScanLineFScope" <- w2943
                "ParametersFScope" <- w2941
                n891 = Unbundle(w2941) -> ("X frequeny [Hz]"=w2936:i32, "Y frequency \n[Hz]"=w2940:i32, "frequeny Trim"=w2937:dbl, "Samples/s"=w2934:i32)  [unwired: 2 out]
                "Pixel Clock (Hz) FScope" <- w2934
                n892 = local write "NewScanpattern"(FALSE ("NewScanpattern")) -> ()
                n893 = Divide(x=w2937, y=200.0) -> (x/y=w2939:dbl)
                n894 = Add(x=w2936, y=w2939) -> (x+y=w2935:dbl)
              }
            }
            n895 = local read "scans to read"() -> (w2848:sgl)
            n896 = Reciprocal(x=w2846) -> (1/x=w2847:dbl)
            n897 = Multiply(x=w2847, y=w2848) -> (x*y=w2845:dbl)
            n898 = Reciprocal(x=w2845) -> (1/x=w2844:dbl)
            n899 = local write "Frame rate [Hz]"(w2844) -> ()
            n900 = case shown="2" w2854 {
              tunnel: [w2877 w2895 w2914] -> w2863
              tunnel: w2853 -> [w2875 w2893 w2913]
              tunnel: [w2868 w2886 w2908] -> w2856
              tunnel: [w2867 w2885 w2907] -> w2855
              tunnel: "LS X/Y" -> [_ _ w2906]
              tunnel: w2851 -> [_ _ w2901]
              tunnel: w2850 -> [_ _ w2899]
              tunnel: w2849 -> [_ _ w2900]
              frame 0, Default {
                w2866 = 10123 items=["Finite Samples"=10178, "Continuous Samples"=10123, "Hardware Timed Single Point"=12522] ("sample mode")
                n901 = Index Array(array=w2875, index (row)=0) -> (element=w2874:dbl[])  [unwired: 1 in]
                n902 = Index Array(array=w2875, index (row)=1) -> (element=w2869:dbl[])  [unwired: 1 in]
                n903 = Add(x=w2874, y=w2869) -> (x+y=w2876:dbl[])
                n904 = Array Max & Min(array=w2874) -> (max value=w2872:dbl, min value=w2873:dbl)  [unwired: 2 out]
                n905 = Array Max & Min(array=w2869) -> (max value=w2870:dbl, min value=w2871:dbl)  [unwired: 2 out]
                n906 = Build Array(w2876) -> (w2877:dbl[][])
                n907 = Array Size(array=w2876) -> (size(s)=w2868:i32)
                n908 = global write "GlobelFSCOPE.vi" "X max"(w2872) -> ()
                n909 = global write "GlobelFSCOPE.vi" "X min"(w2873) -> ()
                n910 = global write "GlobelFSCOPE.vi" "Y max"(w2870) -> ()
                n911 = global write "GlobelFSCOPE.vi" "Y min"(w2871) -> ()
                n912 = Bundle("sample mode"=w2866, "sample mode"=w2866) -> (w2867:cluster{"sample mode":i32, "sample mode":i32})  [unwired: 1 in]
              }
              frame 1 {
                w2880 = 10178 items=["Finite Samples"=10178, "Continuous Samples"=10123, "Hardware Timed Single Point"=12522] ("sample mode")
                n913 = Index Array(array=w2893, index (row)=0) -> (element=w2892:dbl[])  [unwired: 1 in]
                n914 = Index Array(array=w2893, index (row)=1) -> (element=w2887:dbl[])  [unwired: 1 in]
                n915 = Add(x=w2892, y=w2887) -> (x+y=w2894:dbl[])
                n916 = Array Max & Min(array=w2892) -> (max value=w2890:dbl, min value=w2891:dbl)  [unwired: 2 out]
                n917 = Array Max & Min(array=w2887) -> (max value=w2888:dbl, min value=w2889:dbl)  [unwired: 2 out]
                n918 = Build Array(w2894) -> (w2895:dbl[][])
                n919 = Array Size(array=w2894) -> (size(s)=w2886:i32)
                n920 = global write "GlobelFSCOPE.vi" "X max"(w2890) -> ()
                n921 = global write "GlobelFSCOPE.vi" "X min"(w2891) -> ()
                n922 = global write "GlobelFSCOPE.vi" "Y max"(w2888) -> ()
                n923 = global write "GlobelFSCOPE.vi" "Y min"(w2889) -> ()
                n924 = local read "Number of Frames"() -> (w2882:sgl)
                n925 = local read "scans to read"() -> (w2884:sgl)
                n926 = local read "Averaging"() -> (w2883:sgl)
                n927 = Compound Arithmetic op=MULTIPLY(w2884, w2883, w2882) -> (w2881:sgl)
                n928 = Bundle(w2881, "sample mode"=w2880) -> (w2885:cluster{sgl, "sample mode":i32})  [unwired: 1 in]
              }
              frame 2 {
                w2902 = 10123 items=["Finite Samples"=10178, "Continuous Samples"=10123, "Hardware Timed Single Point"=12522] ("sample mode")
                n929 = Index Array(array=w2913, index (row)=0) -> (element=w2905:dbl[])  [unwired: 1 in]
                n930 = Index Array(array=w2913, index (row)=1) -> (element=w2903:dbl[])  [unwired: 1 in]
                n931 = Array Max & Min(array=w2905) -> (max value=w2911:dbl, min value=w2912:dbl)  [unwired: 2 out]
                n932 = Array Max & Min(array=w2903) -> (max value=w2909:dbl, min value=w2910:dbl)  [unwired: 2 out]
                n933 = case shown="False" w2906 {
                  tunnel: [w2920 w2924] -> w2904
                  tunnel: w2905 -> [_ w2924]
                  tunnel: w2903 -> [w2920 _]
                  tunnel: w2901 -> [w2919 w2923]
                  tunnel: w2900 -> [w2918 _]
                  tunnel: w2899 -> [_ w2922]
                  tunnel: [w2917 w2921] -> w2898
                  frame False {
                    n934 = Divide(x=w2919, y=w2918) -> (x/y=w2917:dbl)
                  }
                  frame True {
                    n935 = Divide(x=w2923, y=w2922) -> (x/y=w2921:dbl)
                  }
                }
                n936 = global write "GlobelFSCOPE.vi" "X max"(w2911) -> ()
                n937 = global write "GlobelFSCOPE.vi" "X min"(w2912) -> ()
                n938 = global write "GlobelFSCOPE.vi" "Y max"(w2909) -> ()
                n939 = global write "GlobelFSCOPE.vi" "Y min"(w2910) -> ()
                n940 = local write "scans to read"(w2898) -> ()
                n941 = Build Array(w2904) -> (w2914:dbl[][])
                n942 = Array Size(array=w2904) -> (size(s)=w2908:i32)
                n943 = Bundle("sample mode"=w2902, "sample mode"=w2902) -> (w2907:cluster{"sample mode":i32, "sample mode":i32})  [unwired: 1 in]
              }
            }
            "Scanlength" <- w2856
            n944 = Concatenate Strings(w2858, tag "/ao0" ("physical channels")) -> (w2862:string)
            n945 = Type Cast(type=w2859, x=w2862) -> (*(type *) &x=w2860:tag)
          }
        }
        "ScanSignals" <- w2005
        n946 = Subtract(x=w1879, y=2.0) -> (x-y=w1881:dbl)
        n947 = case shown="True" "Stimulus" {
          tunnel: w1879 -> [_ w2069]
          tunnel: [u32 2 ("low ticks") w2068] -> w1884
          tunnel: [w2062 w2067] -> w1883
          tunnel: [0.0 w2066] -> w1882
          tunnel: w1881 -> [w2062 _]
          tunnel: w1856 -> [_ w2065]
          frame False {
          }
          frame True {
            n948 = Multiply(x="Stimulus Duration [s]", y=sgl 1000000.0) -> (x*y=w2071:sgl)
            n949 = Divide(x=w2071, y=w2065) -> (x/y=w2068:sgl)
            n950 = Multiply(x="Interval [x Lines]", y=w2069) -> (x*y=w2066:dbl)
            n951 = Subtract(x=w2066, y=w2068) -> (x-y=w2067:dbl)
          }
        }
        n952 = call-poly <vilib>:"DAQmx Create Channel (CO-Pulse Generation-Ticks).vi"("high ticks"=w1884, "low ticks"=w1883, "counter"=w1926, "source of ticks"=w1938, "error in"=w1922, "initial delay"=w1882) -> ("task out"=w2022:refnum<k21>, "error out"=w2021:errorcluster)  [unwired: 8 in]
        n953 = property on="Linescan mode" class="Bool (strict)"("Visible"=w1861) -> ()  [unwired: 2 in, 2 out]
        n954 = call-poly <vilib>:"DAQmx Timing (Implicit).vi"("task/channels in"=w2022, "sample mode"=w2020, "error in"=w2021) -> ("task out"=w2019:refnum<k21>, "error out"=w2018:errorcluster)  [unwired: 11 in]
        n955 = Greater Or Equal?(x=w1919, y=u16 1) -> (x >= y?=w1917:bool)
        n956 = call <vilib>:"DAQmx Start Task.vi"("task/channels in"=w2019, "error in"=w2018) -> ("task out"=w1963:refnum<k21>, "error out"=w1924:errorcluster)  [unwired: 12 in]
        n957 = local read "Scangraph scaling"() -> (w1852:sgl)
        n958 = local read "frame/line indicator"() -> (w1921:u16)
        n959 = Multiply(x=w1953, y=w1879) -> (x*y=w1954:dbl)
        n960 = local read "AO/DIO Device"() -> (w1965:tag)
        n961 = local read "Fiberscope\nMode"() -> (w1893:bool)
        n962 = property on="XScale" class="Bool (strict)"("Visible"=w1862) -> ()  [unwired: 2 in, 2 out]
        n963 = property on="Test Run?" class="Bool (strict)"("Visible"=w1862) -> ()  [unwired: 2 in, 2 out]
        n964 = property on="Scale" class="DigNum (strict)"("Visible"=w1862) -> ()  [unwired: 2 in, 2 out]
        n965 = property on="Int Corr?" class="Bool (strict)"("Visible"=w1862) -> ()  [unwired: 2 in, 2 out]
        n966 = Subtract(x=w1954, y=2.0) -> (x-y=w1876:dbl)
        n967 = case shown="True" "Case Constant\n(See Context Help)" {
          tunnel: w1879 -> [_ w2057]
          tunnel: [u32 2 ("low ticks") w2056] -> w1877
          tunnel: [w2050 w2055] -> w1875
          tunnel: [0.0 w2054] -> w1878
          tunnel: w1876 -> [w2050 _]
          tunnel: w1856 -> [_ w2053]
          frame False {
          }
          frame True {
            n968 = Multiply(x="Stimulus Duration [s] 2", y=sgl 1000000.0) -> (x*y=w2059:sgl)
            n969 = Divide(x=w2059, y=w2053) -> (x/y=w2056:sgl)
            n970 = Multiply(x="Interval [x Lines] 2", y=w2057) -> (x*y=w2054:dbl)
            n971 = Subtract(x=w2054, y=w2056) -> (x-y=w2055:dbl)
          }
        }
        n972 = Array Subset(array=w2005, length (row)=2 ("length")) -> (w2004:dbl[][])  [unwired: 3 in]
        n973 = local read "AO/DIO Device"() -> (w1928:tag)
        n974 = Concatenate Strings(w1965, tag "/port0" ("lines")) -> (w1973:string)
        n975 = Array Max & Min(array=w2004) -> (max value=w2007:dbl, min value=w2006:dbl)  [unwired: 2 out]
        n976 = local read "AO/DIO Device"() -> (w1934:tag)
        n977 = Decrement(x=w1852) -> (x-1=w1854:sgl)
        n978 = Equal To 0?(x=w1921) -> (x = 0?=w1920:bool)
        n979 = case shown="True" w1893 {
          tunnel: [w2075 w2078] -> w2027
          tunnel: w1920 -> [w2074 _]
          frame False {
            n980 = case shown="False" w2074 {
              tunnel: [w2076 w2077] -> w2075
              frame False {
                w2076 = 10097 items=["Allow Regeneration"=10097, "Do Not Allow Regeneration"=10158] ("RegenMode")
              }
              frame True {
                w2077 = 10158 items=["Allow Regeneration"=10097, "Do Not Allow Regeneration"=10158] ("RegenMode")
              }
            }
          }
          frame True {
            w2078 = 10097 items=["Allow Regeneration"=10097, "Do Not Allow Regeneration"=10158] ("RegenMode")
          }
        }
        n981 = Type Cast(type=tag "" ("lines"), x=w1973) -> (*(type *) &x=w1970:tag)
        n982 = Negate(x=w1854) -> (-x=w1855:sgl)
        n983 = Negate(x=w1852) -> (-x=w1853:sgl)
        n984 = In Range and Coerce(upper limit=10.0 ("y"), x=w1888, lower limit=-10.0 ("y")) -> (coerced(x)=w1889:dbl[][])  [unwired: 1 out]
        n985 = local read "AO/DIO Device"() -> (w1913:tag)
        n986 = Concatenate Strings(tag "/" ("destination terminal"), w1913) -> (w1907:string)
        n987 = Concatenate Strings(tag "/" ("destination terminal"), w1928, tag "/ao/SampleClock" ("source of ticks")) -> (w1933:string)
        n988 = call-poly <vilib>:"DAQmx Create Channel (DI-Digital Input).vi"("lines"=w1970, "error in"=w1922) -> ("task out"=w1952:refnum<k21>, "error out"=w1950:errorcluster)  [unwired: 12 in]
        n989 = Index Array(array=w2004, index (row)=1 ("index")) -> (element=w2041:dbl[])  [unwired: 1 in]
        n990 = Concatenate Strings(w1934, tag "/ctr1" ("counter")) -> (w1936:string)
        n991 = Concatenate Strings(tag "/" ("destination terminal"), w1965, tag "/ao/SampleClock" ("source terminal")) -> (w1969:string)
        n992 = Greater?(x=w2007, y=w1854) -> (0:w2045:bool)
        n993 = Less?(x=w2006, y=w1855) -> (x < y?=w2046:bool)
        n994 = Type Cast(type=tag "" ("source of ticks"), x=w1933) -> (*(type *) &x=w1929:tag)
        n995 = Or(x=w2045, y=w2046) -> (x .or. y?=w2043:bool)
        n996 = Index Array(array=w2004, index (row)=0 ("index")) -> (element=w2040:dbl[])  [unwired: 1 in]
        n997 = Type Cast(type=tag "" ("counter"), x=w1936) -> (*(type *) &x=w1935:tag)
        n998 = Type Cast(type=tag "" ("source terminal"), x=w1969) -> (*(type *) &x=w1964:tag)
        n999 = Concatenate Strings(tag "/" ("destination terminal"), w1913) -> (w1897:string)
        n1000 = case shown="True" w2043 {
          tunnel: [u32 0 w3030] -> w2042
          tunnel: w2004 -> [_ w3025]
          tunnel: w1853 -> [_ w3023]
          tunnel: w1852 -> [_ w3022]
          frame False {
          }
          frame True {
